vi "IND560 Serial FGV Filter.vi"(8 "Error In":errorcluster, 10 "Bytes at Port":u32, 11 "Weight Template":string) -> (0 "Error Out":errorcluster, 3 "Filtered Weight":string)   [LabVIEW 2023]
uses:
  <vilib>/Utility/error.llb/whitespace.ctl
  <vilib>/Utility/error.llb/Trim Whitespace One-Sided.vi
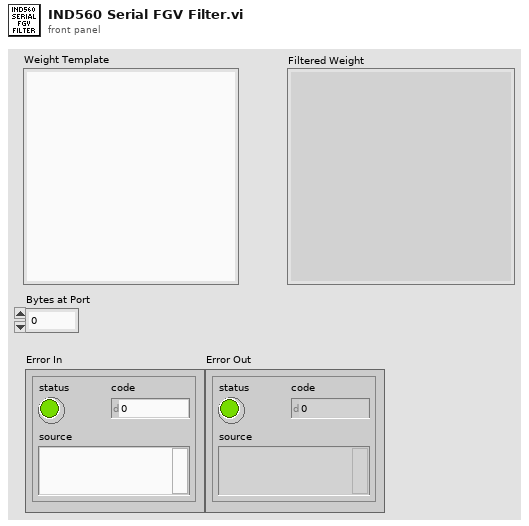
[diagram p1: front panel]
types:
  T1 = typedef "whitespace.ctl" = u16
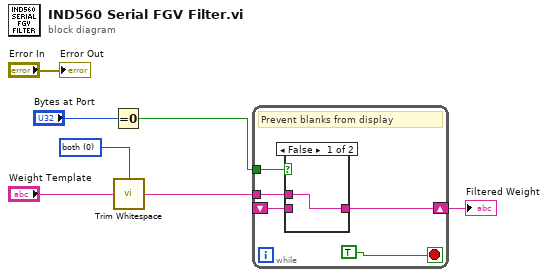
[diagram p0: block diagram]
diagram:
  w5 = T1 0 items=["both", "start of string", "end of string"] ("location (both)")
  n1 = Equal To 0?(x="Bytes at Port") -> (x = 0?=w6:bool)
  n2 = call <vilib>:"Trim Whitespace.vi"("string"="Weight Template", "location (both)"=w5) -> ("trimmed string"=w1:string)
  n3 = while {
    tunnel: w6 -> [w12]
    tunnel: w1 -> [w10]
    shift-right: [w9] -> w7
    shift-left: _ -> [w11]
    stop <- TRUE stop-if-true
    # "Prevent blanks from display"
    n4 = case shown="False" w12 {
      tunnel: w11 -> [_ w14]
      tunnel: w10 -> [w13 _]
      tunnel: [w13 w14] -> w9
      frame False {
      }
      frame True {
      }
    }
  }
  "Filtered Weight" <- w7
  "Error Out" <- "Error In"
